vi "niScope Clear Error Info.vi"(0 "instrument handle":refnum<k15>, 11 "error in":errorcluster) -> (4 "instrument handle out":refnum<k15>, 15 "error out":errorcluster)   [LabVIEW 2013]
doc: "Clears the error information for the current execution thread and the IVI session you specify. If you pass VI_NULL for the Instrument Handle, this VI clears the error information only for the current execution thread."
uses:
  niScope_32.dll
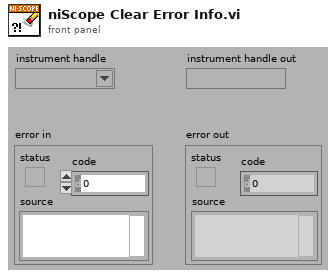
[diagram p1: front panel]
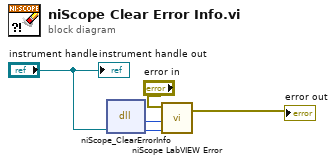
[diagram p0: block diagram]
diagram:
  n1 = dll-call lib="niScope_*.*" fn="niScope_ClearErrorInfo"("instrument handle"="instrument handle") -> ("status"=w4:i32, "instrument handle"=w3:u32)  [unwired: 3 in, 2 out]
  n2 = call <instrlib>:"niScope LabVIEW Error.vi"("instrument handle"=w3, "niScope error code (0)"=w4, "error in (no error)"="error in") -> ("error out"=→"error out":errorcluster)  [unwired: 2 in]
  "instrument handle out" <- "instrument handle"
